vi "Begin.vi"() -> (0 "error out":errorcluster)   [LabVIEW 2017]
doc: "Called before other user functions, this VI is expected to open initial I/O refnums, load in file data, and do all program initialization. Notice that the <B>error out</B> terminal is simply used for data flow. Wiring it to other structures or subVIs ensures that this VI runs first."
uses:
  Public/Documents/Cross The Road Electronics/Phoenix-LabVIEW/Motor Controller/Controls/CTRE_Phoenix_MotorControl_NeutralMode.ctl
  Public/Documents/Cross The Road Electronics/Phoenix-LabVIEW/Motor Controller/Controls/CTRE_Phoenix_MotorControl_FeedbackDevice.ctl
  <vilib>/Rock Robotics/WPI/Joystick/WPI_JoystickDeviceEnum.ctl
  <vilib>/Rock Robotics/WPI/RobotDrive/WPI_RobotDriveOpen2MotorWithSPARK.vi
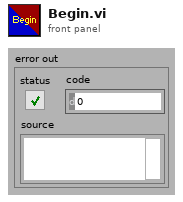
[diagram p1: front panel]
types:
  T1 = typedef "CTRE_Phoenix_MotorControl_FeedbackDevice.ctl" = i8
  T2 = typedef "CTRE_Phoenix_MotorControl_NeutralMode.ctl" = enum8{"EEPROMSetting", "Override to Coast", "Override to Brake"}
  T3 = typedef "WPI_JoystickDeviceEnum.ctl" = enum16{"USB 0", "USB 1", "USB 2", "USB 3", "USB 4", "USB 5"}
  T4 = typedef "WPI_MotorControlDeviceRef.ctl" = cluster{"DeviceStatus":errorcluster, "Type":T5, "PWM":cluster{"PWM Channel":T6, "DeadBand":T7}, "CAN":cluster{"Device Number":u8, "SetOutput VI Ref":variant, "GetOutput VI Ref":variant, "Enable VI Ref":variant, "Disable VI Ref":variant, "Data":variant}, "Invert":bool, "DIO PWM":cluster{"PWM \"Enable\" Channel":T6, "DIOChannel":T8, "PWM Rate":dbl}}
  T5 = typedef "WPI_MotorControlType.ctl" = enum16{"PWM", "CAN", "DIO PWM"}
  T6 = typedef "FPGA_DIOPWMChannel.ctl" = enum8{"PWM 0", "PWM 1", "PWM 2", "PWM 3", "PWM 4", "PWM 5", "PWM 6", "PWM 7", "PWM 8", "PWM 9", "PWM MXP 0", "PWM MXP 1", "PWM MXP 2", "PWM MXP 3", "PWM MXP 4", "PWM MXP 5", "PWM MXP 6", "PWM MXP 7", "PWM MXP 8", "PWM MXP 9", "Invalid"}
  T7 = typedef "WPI_PWMDeadband.ctl" = cluster{"Name":string, "maxPositivePwm":i32, "minPositivePwm":i32, "centerPwm":i32, "maxNegativePwm":i32, "minNegativePwm":i32, "angularRange":u16}
  T8 = typedef "FPGA_DIOChannel.ctl" = enum8{"DIO 0", "DIO 1", "DIO 2", "DIO 3", "DIO 4", "DIO 5", "DIO 6", "DIO 7", "DIO 8", "DIO 9", "DIO MXP 0", "DIO MXP 1", "DIO MXP 2", "DIO MXP 3", "DIO MXP 4", "DIO MXP 5", "DIO MXP 6", "DIO MXP 7", "DIO MXP 8", "DIO MXP 9", "DIO MXP 10", "DIO MXP 11", "DIO MXP 12", "DIO MXP 13", "DIO MXP 14", "DIO MXP 15", "SPI Port CS1", "SPI Port CS2", "SPI Port CS3", "SPI Port MISO", "SPI Port MOSI", "Invalid"}
  T9 = typedef "WPI_JoystickDevRef.ctl" = cluster{"Device":T3}
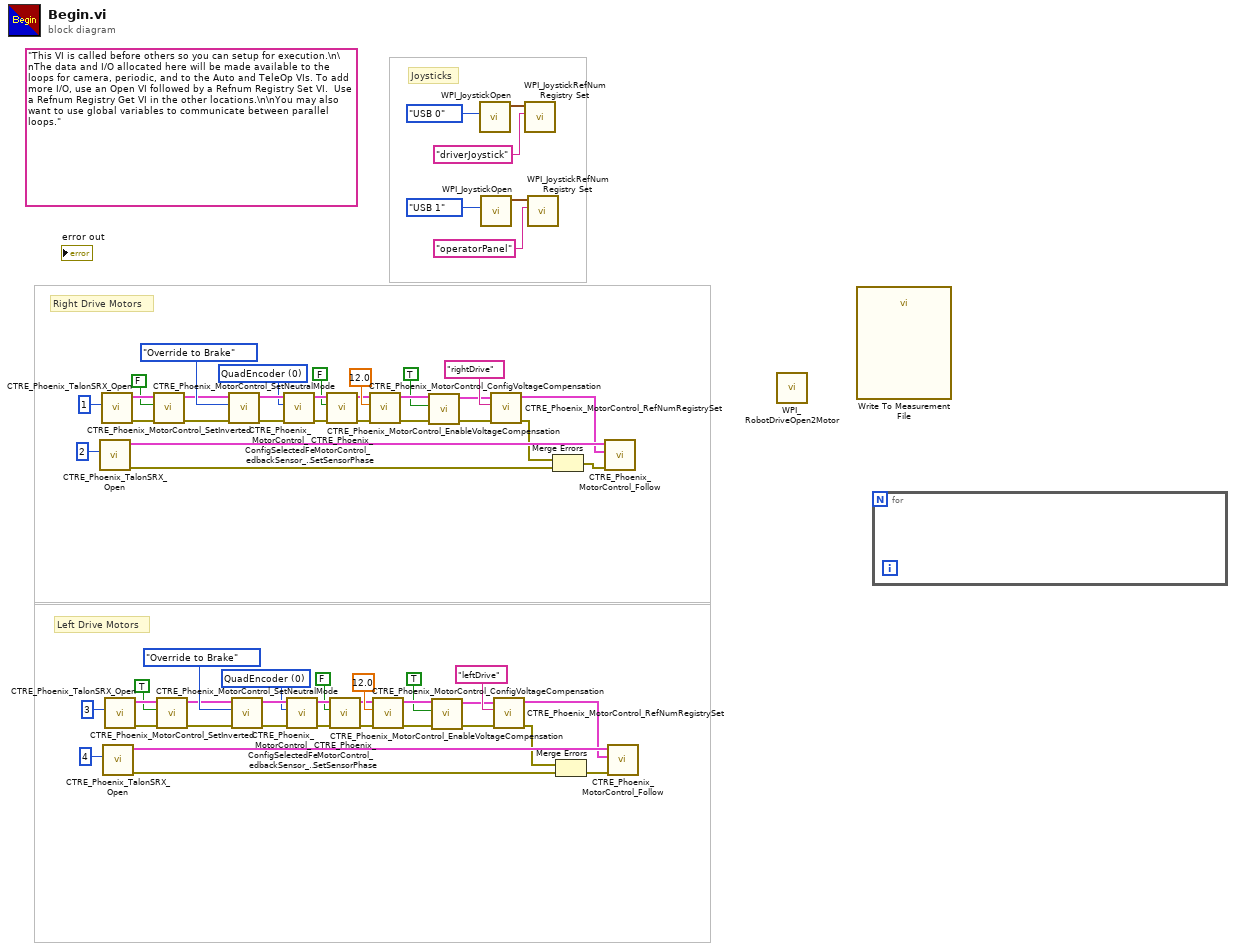
[diagram p0: block diagram]
diagram:
  w7 = T1 0 items=["None"=-1, "QuadEncoder"=0, "Analog"=2, "Tachometer"=4, "Pulse Width Encoded Position"=8, "Sensor Sum (S0 + S1)"=9, "Sensor Difference (D0 - D1)"=10, "Remote Source 0"=11, "Remote Source 1"=12, "Software Emulated"=15] ("Feedback Device")
  w41 = T1 0 items=["None"=-1, "QuadEncoder"=0, "Analog"=2, "Tachometer"=4, "Pulse Width Encoded Position"=8, "Sensor Sum (S0 + S1)"=9, "Sensor Difference (D0 - D1)"=10, "Remote Source 0"=11, "Remote Source 1"=12, "Software Emulated"=15] ("Feedback Device")
  (unwired) "This VI is called before others so you can setup for execution.\n\nThe data and I/O allocated here will be made available to the loops for camera, periodic, and to the Auto and TeleOp VIs. To add more I/O, use an Open VI followed by a Refnum Registry Set VI.  Use a Refnum Registry Get VI in the other locations.\n\nYou may also want to use global variables to communicate between parallel loops."
  # "Joysticks"
  # "Left Drive Motors"
  # "Right Drive Motors"
  n1 = call "CTRE_Phoenix_TalonSRX_Open.vi"("Device Number"=u8 2) -> ("error out"=w51:errorcluster, "CAN Talon SRX Ref"=w59:T4)  [unwired: 9 in]
  n2 = call "CTRE_Phoenix_TalonSRX_Open.vi"("Device Number"=u8 1) -> ("error out"=w30:errorcluster, "CAN Talon SRX Ref"=w31:T4)  [unwired: 9 in]
  n3 = call "CTRE_Phoenix_TalonSRX_Open.vi"("Device Number"=u8 4) -> ("error out"=w17:errorcluster, "CAN Talon SRX Ref"=w25:T4)  [unwired: 9 in]
  n4 = call "CTRE_Phoenix_TalonSRX_Open.vi"("Device Number"=u8 3) -> ("error out"=w2:errorcluster, "CAN Talon SRX Ref"=w3:T4)  [unwired: 9 in]
  n5 = call "CTRE_Phoenix_MotorControl_SetInverted.vi"("error in (no error)"=w30, "Invert?"=FALSE, "PhoenixMotorControlDevRef"=w31) -> ("error out"=w33:errorcluster, "PhoenixMotorControlDevRef"=w32:T4)  [unwired: 7 in]
  n6 = call "CTRE_Phoenix_MotorControl_SetInverted.vi"("error in (no error)"=w2, "Invert?"=TRUE, "PhoenixMotorControlDevRef"=w3) -> ("error out"=w5:errorcluster, "PhoenixMotorControlDevRef"=w4:T4)  [unwired: 7 in]
  n7 = call "CTRE_Phoenix_MotorControl_SetNeutralMode.vi"("error in (no error)"=w33, "Motor Control Neutral Mode"=CTRE_Phoenix_MotorControl_NeutralMode."Override to Brake", "PhoenixMotorControlDevRef"=w32) -> ("error out"=w57:errorcluster, "PhoenixMotorControlDevRef"=w58:T4)  [unwired: 7 in]
  n8 = call "CTRE_Phoenix_MotorControl_SetNeutralMode.vi"("error in (no error)"=w5, "Motor Control Neutral Mode"=CTRE_Phoenix_MotorControl_NeutralMode."Override to Brake", "PhoenixMotorControlDevRef"=w4) -> ("error out"=w23:errorcluster, "PhoenixMotorControlDevRef"=w24:T4)  [unwired: 7 in]
  n9 = call "CTRE_Phoenix_MotorControl_ConfigSelectedFeedbackSensor_Enhanced.vi"("error in (no error)"=w57, "Feedback Device"=w41, "PhoenixMotorControlDevRef"=w58) -> ("error out"=w54:errorcluster, "PhoenixMotorControlDevRef"=w55:T4)  [unwired: 7 in]
  n10 = call "CTRE_Phoenix_MotorControl_ConfigSelectedFeedbackSensor_Enhanced.vi"("error in (no error)"=w23, "Feedback Device"=w7, "PhoenixMotorControlDevRef"=w24) -> ("error out"=w20:errorcluster, "PhoenixMotorControlDevRef"=w21:T4)  [unwired: 7 in]
  n11 = call "CTRE_Phoenix_MotorControl_SetSensorPhase.vi"("error in (no error)"=w54, "PhaseSensor"=FALSE, "PhoenixMotorControlDevRef"=w55) -> ("error out"=w47:errorcluster, "PhoenixMotorControlDevRef"=w48:T4)  [unwired: 7 in]
  n12 = call "CTRE_Phoenix_MotorControl_SetSensorPhase.vi"("error in (no error)"=w20, "PhaseSensor"=FALSE, "PhoenixMotorControlDevRef"=w21) -> ("error out"=w13:errorcluster, "PhoenixMotorControlDevRef"=w14:T4)  [unwired: 7 in]
  n13 = call "CTRE_Phoenix_MotorControl_ConfigVoltageCompensation.vi"("error in (no error)"=w47, "Saturation Voltage"=12.0, "PhoenixMotorControlDevRef"=w48) -> ("error out"=w45:errorcluster, "PhoenixMotorControlDevRef"=w46:T4)  [unwired: 7 in]
  n14 = call "CTRE_Phoenix_MotorControl_ConfigVoltageCompensation.vi"("error in (no error)"=w13, "Saturation Voltage"=12.0, "PhoenixMotorControlDevRef"=w14) -> ("error out"=w11:errorcluster, "PhoenixMotorControlDevRef"=w12:T4)  [unwired: 7 in]
  n15 = call "CTRE_Phoenix_MotorControl_EnableVoltageCompensation.vi"("error in (no error)"=w45, "Enable Voltage Compensation?"=TRUE, "PhoenixMotorControlDevRef"=w46) -> ("error out"=w42:errorcluster, "PhoenixMotorControlDevRef"=w43:T4)  [unwired: 7 in]
  n16 = call "CTRE_Phoenix_MotorControl_EnableVoltageCompensation.vi"("error in (no error)"=w11, "Enable Voltage Compensation?"=TRUE, "PhoenixMotorControlDevRef"=w12) -> ("error out"=w8:errorcluster, "PhoenixMotorControlDevRef"=w9:T4)  [unwired: 7 in]
  n17 = call <vilib>:"WPI_JoystickOpen.vi"("JoystickDevice"=WPI_JoystickDeviceEnum."USB 0") -> ("JoystickDevRef"=w39:T9)  [unwired: 10 in]
  n18 = call <vilib>:"WPI_JoystickOpen.vi"("JoystickDevice"=WPI_JoystickDeviceEnum."USB 1") -> ("JoystickDevRef"=w36:T9)  [unwired: 10 in]
  n19 = call "CTRE_Phoenix_MotorControl_RefNumRegistrySet.vi"("error in (no error)"=w42, "refnum name"="rightDrive", "PhoenixMotorControlDevRef"=w43) -> ("error out"=w50:errorcluster, "PhoenixMotorControlDevRef"=w40:T4)  [unwired: 7 in]
  n20 = call "CTRE_Phoenix_MotorControl_RefNumRegistrySet.vi"("error in (no error)"=w8, "refnum name"="leftDrive", "PhoenixMotorControlDevRef"=w9) -> ("error out"=w16:errorcluster, "PhoenixMotorControlDevRef"=w6:T4)  [unwired: 7 in]
  n21 = call <vilib>:"WPI_JoystickRefNum Registry Set.vi"("refnum name"="driverJoystick", "JoystickDevRef"=w39) -> ()  [unwired: 8 in, 2 out]
  n22 = call <vilib>:"WPI_JoystickRefNum Registry Set.vi"("refnum name"="operatorPanel", "JoystickDevRef"=w36) -> ()  [unwired: 8 in, 2 out]
  n23 = Merge Errors(w50, w51) -> (w52:errorcluster)
  n24 = Merge Errors(w16, w17) -> (w18:errorcluster)
  n25 = call "CTRE_Phoenix_MotorControl_Follow.vi"("error in (no error)"=w52, "Master Controller to Follow"=w40, "PhoenixMotorControlDevRef"=w59) -> ()  [unwired: 7 in, 2 out]
  n26 = call "CTRE_Phoenix_MotorControl_Follow.vi"("error in (no error)"=w18, "Master Controller to Follow"=w6, "PhoenixMotorControlDevRef"=w25) -> ()  [unwired: 7 in, 2 out]
  n27 = call-poly <vilib>:"WPI_RobotDriveOpen2Motor.vi"() -> ()  [unwired: 10 in, 2 out]
  n28 = call "Write To Measurement File"() -> ()  [unwired: 17 in, 3 out]
  n29 = for {
  }
